vi "log analysis_gps.vi"() -> ()   [LabVIEW 2018] (continued)
0.0963,0.1004,5.0820,0f000001,0*f4eeef52\n\t", "INSPVAXA,USB3,0,47.5,FINESTEERING,2107,283761.800,02000000,471d,15824;INS_ALIGNMENT_COMPLETE,INS_RTKFIXED,37.37107239859,126.72171850723,8.1174,22.3000,-0.3618,-0.2694,0.0247,-0.806586304,0.185409278,212.363938082,0.4339,0.3017,0.5874,0.1136,0.0941,0.0830,0.0963,0.1004,5.0820,0f000001,0*fafaa8b9\n\t", "INSPVAXA,USB3,0,49.5,FINESTEERING,2107,283762.300,02000000,471d,15824;INS_ALIGNMENT_COMPLETE,INS_RTKFIXED,37.37107064339,126.72171694758,8.1181,22.3000,-0.3599,-0.2839,0.0222,-0.849299208,0.007344260,212.586929026,0.4338,0.3017,0.5881,0.1135,0.0943,0.0833,0.0964,0.1005,5.0831,0f000001,0*fde6b9b2\n\t", "DUALANTENNAHEADINGA,USB3,0,49.5,FINESTEERING,2107,283762.800,02000000,d426,15824;INSUFFICIENT_OBS,NONE,-1.000000000,0.000000000,0.000000000,0.0,0.000000000,0.000000000,\"631T\",11,2,2,2,04,00,20,00*344581c2\n\t", "INSPVAXA,USB3,0,49.5,FINESTEERING,2107,283763.300,02000000,471d,15824;INS_ALIGNMENT_COMPLETE,INS_RTKFIXED,37.37106722577,126.72171383567,8.1242,22.3000,-0.3707,-0.2828,0.0344,-0.877287415,-0.329953157,212.884392391,0.4341,0.3014,0.5889,0.1138,0.0946,0.0836,0.0965,0.1006,5.0839,0f000001,0*2db501e2\n\t", "INSPVAXA,USB3,0,49.5,FINESTEERING,2107,283763.800,02000000,471d,15824;INS_ALIGNMENT_COMPLETE,INS_RTKFIXED,37.37106551581,126.72171225128,8.1242,22.3000,-0.3497,-0.2822,0.0044,-0.644975976,-0.227422020,213.086413848,0.4341,0.3014,0.5889,0.1138,0.0946,0.0836,0.0965,0.1006,5.0839,0f000001,0*e7a51fd5\n\t", "INSPVAXA,USB3,0,50.0,FINESTEERING,2107,283764.300,02000000,471d,15824;INS_ALIGNMENT_COMPLETE,INS_RTKFIXED,37.37106379034,126.72171067271,8.1222,22.3000,-0.3531,-0.2829,0.0306,-0.817396197,-0.204433431,213.191870760,0.4344,0.3013,0.5897,0.1145,0.0953,0.0847,0.0966,0.1006,5.0845,0f000001,0*c35694b0\n\t", "INSPVAXA,USB3,0,50.0,FINESTEERING,2107,283764.800,02000000,471d,15824;INS_ALIGNMENT_COMPLETE,INS_RTKFIXED,37.37106210013,126.72170911188,8.1232,22.3000,-0.3512,-0.2846,0.0354,-0.878103846,0.017122797,213.188721115,0.4344,0.3013,0.5897,0.1145,0.0953,0.0847,0.0966,0.1006,5.0845,0f000001,0*f1b4f4ee\n\t", "INSPVAXA,USB3,0,48.5,FINESTEERING,2107,283765.300,02000000,471d,15824;INS_ALIGNMENT_COMPLETE,INS_RTKFIXED,37.37106036944,126.72170751159,8.1232,22.3000,-0.3518,-0.2906,0.0186,-0.822067301,0.160317962,213.455699651,0.4347,0.3015,0.5906,0.1149,0.0956,0.0855,0.0967,0.1007,5.0850,0f000001,0*76086230\n\t", "INSPVAXA,USB3,0,48.5,FINESTEERING,2107,283765.800,02000000,471d,15824;INS_ALIGNMENT_COMPLETE,INS_RTKFIXED,37.37105862901,126.72170591999,8.1228,22.3000,-0.3574,-0.2825,0.0115,-1.119312429,-0.040061536,213.743406523,0.4347,0.3015,0.5906,0.1149,0.0956,0.0855,0.0967,0.1007,5.0850,0f000001,0*ba4559e2\n\t", "INSPVAXA,USB3,0,49.5,FINESTEERING,2107,283766.300,02000000,471d,15824;INS_ALIGNMENT_COMPLETE,INS_RTKFIXED,37.37105695228,126.72170433159,8.1249,22.3000,-0.3688,-0.2983,0.0300,-0.908838629,-0.130495900,213.736346026,0.4351,0.3021,0.5917,0.1155,0.0961,0.0864,0.0968,0.1008,5.0859,0f000001,0*b472baf5\n\t", "DUALANTENNAHEADINGA,USB3,0,49.5,FINESTEERING,2107,283766.800,02000000,d426,15824;INSUFFICIENT_OBS,NONE,-1.000000000,0.000000000,0.000000000,0.0,0.000000000,0.000000000,\"631T\",12,2,2,2,04,00,20,00*fb02124e\n\t", "INSPVAXA,USB3,0,42.5,FINESTEERING,2107,283767.300,02000000,471d,15824;INS_ALIGNMENT_COMPLETE,INS_RTKFIXED,37.37105380440,126.72170132939,8.1248,22.3000,-0.4012,-0.3058,0.0222,-0.759918360,0.196787638,213.771684261,0.4356,0.3025,0.5930,0.1157,0.0960,0.0864,0.0969,0.1009,5.0866,0f000001,0*582355d6\n\t", "DUALANTENNAHEADINGA,USB3,0,42.5,FINESTEERING,2107,283767.800,02000000,d426,15824;INSUFFICIENT_OBS,NONE,-1.000000000,0.000000000,0.000000000,0.0,0.000000000,0.000000000,\"631T\",11,2,2,2,04,00,20,00*0d855270\n\t", "DUALANTENNAHEADINGA,USB3,0,49.5,FINESTEERING,2107,283768.300,02000000,d426,15824;INSUFFICIENT_OBS,NONE,-1.000000000,0.000000000,0.000000000,0.0,0.000000000,0.000000000,\"631T\",13,2,2,2,04,00,20,00*d65186ff\n\t", "INSPVAXA,USB3,0,49.5,FINESTEERING,2107,283768.800,02000000,471d,15824;INS_ALIGNMENT_COMPLETE,INS_RTKFIXED,37.37104867092,126.72169640975,8.1299,22.3000,-0.3630,-0.2854,0.0072,-0.696189759,0.706458627,213.919013530,0.4366,0.3037,0.5940,0.1145,0.0950,0.0854,0.0970,0.1010,5.0873,0f000001,0*a94daabe\n\t", "DUALANTENNAHEADINGA,USB3,0,49.0,FINESTEERING,2107,283769.300,02000000,d426,15824;INSUFFICIENT_OBS,NONE,-1.000000000,0.000000000,0.000000000,0.0,0.000000000,0.000000000,\"631T\",11,2,2,2,04,00,20,00*9a47621b\n\t", "INSPVAXA,USB3,0,49.0,FINESTEERING,2107,283769.800,02000000,471d,15824;INS_ALIGNMENT_COMPLETE,INS_RTKFIXED,37.37104525737,126.72169313095,8.1331,22.3000,-0.3548,-0.2589,0.0390,-0.749813070,0.572311932,213.822472384,0.4366,0.3042,0.5948,0.1140,0.0941,0.0845,0.0971,0.1011,5.0877,0f000001,0*7155f04b\n\t", "DUALANTENNAHEADINGA,USB3,0,51.5,FINESTEERING,2107,283770.300,02000000,d426,15824;INSUFFICIENT_OBS,NONE,-1.000000000,0.000000000,0.000000000,0.0,0.000000000,0.000000000,\"631T\",11,2,2,2,04,00,20,00*c0be82b5\n\t", "INSPVAXA,USB3,0,51.5,FINESTEERING,2107,283770.800,02000000,471d,15824;INS_ALIGNMENT_COMPLETE,INS_RTKFIXED,37.37104183450,126.72168993931,8.1368,22.3000,-0.3882,-0.2885,0.0511,-0.819164029,0.307516515,213.418856918,0.4363,0.3032,0.5950,0.1136,0.0937,0.0835,0.0972,0.1011,5.0881,0f000001,0*aed1500e\n\t", "INSPVAXA,USB3,0,48.5,FINESTEERING,2107,283771.300,02000000,471d,15824;INS_ALIGNMENT_COMPLETE,INS_RTKFIXED,37.37104011891,126.72168833768,8.1396,22.3000,-0.3597,-0.2669,0.0230,-0.734280477,0.363827676,213.144857898,0.4357,0.3026,0.5950,0.1131,0.0936,0.0827,0.0973,0.1011,5.0881,0f000001,0*55c65246\n\t", "DUALANTENNAHEADINGA,USB3,0,48.5,FINESTEERING,2107,283771.800,02000000,d426,15824;INSUFFICIENT_OBS,NONE,-1.000000000,0.000000000,0.000000000,0.0,0.000000000,0.000000000,\"631T\",12,2,2,2,04,00,20,00*ba5d6ed0\n\t", "DUALANTENNAHEADINGA,USB3,0,51.5,FINESTEERING,2107,283772.300,02000000,d426,15824;INSUFFICIENT_OBS,NONE,-1.000000000,0.000000000,0.000000000,0.0,0.000000000,0.000000000,\"631T\",10,2,2,2,04,00,20,00*ccec0b5f\n\t", "DUALANTENNAHEADINGA,USB3,0,51.5,FINESTEERING,2107,283772.800,02000000,d426,15824;INSUFFICIENT_OBS,NONE,-1.000000000,0.000000000,0.000000000,0.0,0.000000000,0.000000000,\"631T\",11,2,2,2,04,00,20,00*8e3ca933\n\t", "DUALANTENNAHEADINGA,USB3,0,51.0,FINESTEERING,2107,283773.300,02000000,d426,15824;INSUFFICIENT_OBS,NONE,-1.000000000,0.000000000,0.000000000,0.0,0.000000000,0.000000000,\"631T\",11,2,2,2,04,00,20,00*23ac6912\n\t", "DUALANTENNAHEADINGA,USB3,0,51.0,FINESTEERING,2107,283773.800,02000000,d426,15824;INSUFFICIENT_OBS,NONE,-1.000000000,0.000000000,0.000000000,0.0,0.000000000,0.000000000,\"631T\",11,2,2,2,04,00,20,00*b69e4b26\n\t", "DUALANTENNAHEADINGA,USB3,0,51.5,FINESTEERING,2107,283774.300,02000000,d426,15824;INSUFFICIENT_OBS,NONE,-1.000000000,0.000000000,0.000000000,0.0,0.000000000,0.000000000,\"631T\",10,2,2,2,04,00,20,00*7b4d17c8\n\t", "DUALANTENNAHEADINGA,USB3,0,51.5,FINESTEERING,2107,283774.800,02000000,d426,15824;INSUFFICIENT_OBS,NONE,-1.000000000,0.000000000,0.000000000,0.0,0.000000000,0.000000000,\"631T\",9,2,2,2,04,00,20,00*16022d9f\n\t", "INSPVAXA,USB3,0,52.5,FINESTEERING,2107,283775.300,02000000,471d,15824;INS_ALIGNMENT_COMPLETE,INS_RTKFIXED,37.37102638218,126.72167583323,8.1427,22.3000,-0.3501,-0.2557,0.0203,-0.739090378,0.635309618,211.720087902,0.4333,0.3004,0.5913,0.1131,0.0941,0.0802,0.0969,0.1010,5.0876,0f000001,0*37c46ea0\n\t", "INSPVAXA,USB3,0,52.5,FINESTEERING,2107,283775.800,02000000,471d,15824;INS_ALIGNMENT_COMPLETE,INS_RTKFIXED,37.37102462935,126.72167425219,8.1431,22.3000,-0.3596,-0.2647,0.0054,-0.635685510,0.684071691,211.684016338,0.4333,0.3004,0.5913,0.1131,0.0941,0.0802,0.0969,0.1010,5.0876,0f000001,0*5c9971d0\n\t", "DUALANTENNAHEADINGA,USB3,0,52.0,FINESTEERING,2107,283776.300,02000000,d426,15824;INSUFFICIENT_OBS,NONE,-1.000000000,0.000000000,0.000000000,0.0,0.000000000,0.000000000,\"631T\",11,2,2,2,04,00,20,00*8ea80302\n\t", "INSPVAXA,USB3,0,52.0,FINESTEERING,2107,283776.800,02000000,471d,15824;INS_ALIGNMENT_COMPLETE,INS_RTKFIXED,37.37102123220,126.72167119947,8.1450,22.3000,-0.3884,-0.2739,0.0352,-0.693294661,0.196719454,211.670955627,0.4336,0.3004,0.5905,0.1143,0.0952,0.0818,0.0967,0.1009,5.0864,0f000001,0*acb72d28\n\t", "DUALANTENNAHEADINGA,USB3,0,49.0,FINESTEERING,2107,283777.300,02000000,d426,15824;INSUFFICIENT_OBS,NONE,-1.000000000,0.000000000,0.000000000,0.0,0.000000000,0.000000000,\"631T\",10,2,2,2,04,00,20,00*dd4466ea\n\t", "INSPVAXA,USB3,0,49.0,FINESTEERING,2107,283777.800,02000000,471d,15824;INS_ALIGNMENT_COMPLETE,INS_RTKFIXED,37.37101775976,126.72166805938,8.1480,22.3000,-0.3623,-0.2643,0.0243,-0.564736999,0.528719086,211.738950079,0.4339,0.3012,0.5898,0.1140,0.0954,0.0814,0.0965,0.1008,5.0862,0f000001,0*673a0e61\n\t", "DUALANTENNAHEADINGA,USB3,0,52.0,FINESTEERING,2107,283778.300,02000000,d426,15824;INSUFFICIENT_OBS,NONE,-1.000000000,0.000000000,0.000000000,0.0,0.000000000,0.000000000,\"631T\",10,2,2,2,04,00,20,00*36c9b587\n\t", "DUALANTENNAHEADINGA,USB3,0,52.0,FINESTEERING,2107,283778.800,02000000,d426,15824;INSUFFICIENT_OBS,NONE,-1.000000000,0.000000000,0.000000000,0.0,0.000000000,0.000000000,\"631T\",12,2,2,2,04,00,20,00*d74f9142\n\t", "DUALANTENNAHEADINGA,USB3,0,51.0,FINESTEERING,2107,283779.300,02000000,d426,15824;INSUFFICIENT_OBS,NONE,-1.000000000,0.000000000,0.000000000,0.0,0.000000000,0.000000000,\"631T\",11,2,2,2,04,00,20,00*203e4aea\n\t", "DUALANTENNAHEADINGA,USB3,0,51.0,FINESTEERING,2107,283779.800,02000000,d426,15824;INSUFFICIENT_OBS,NONE,-1.000000000,0.000000000,0.000000000,0.0,0.000000000,0.000000000,\"631T\",11,2,2,2,04,00,20,00*b50c68de\n\t", "DUALANTENNAHEADINGA,USB3,0,51.0,FINESTEERING,2107,283780.300,02000000,d426,15824;INSUFFICIENT_OBS,NONE,-1.000000000,0.000000000,0.000000000,0.0,0.000000000,0.000000000,\"631T\",11,2,2,2,04,00,20,00*92abfb52\n\t", "DUALANTENNAHEADINGA,USB3,0,51.0,FINESTEERING,2107,283780.800,02000000,d426,15824;INSUFFICIENT_OBS,NONE,-1.000000000,0.000000000,0.000000000,0.0,0.000000000,0.000000000,\"631T\",13,2,2,2,04,00,20,00*732ddf97\n\t", "DUALANTENNAHEADINGA,USB3,0,48.5,FINESTEERING,2107,283781.300,02000000,d426,15824;INSUFFICIENT_OBS,NONE,-1.000000000,0.000000000,0.000000000,0.0,0.000000000,0.000000000,\"631T\",13,2,2,2,04,00,20,00*ffe25397\n\t", "DUALANTENNAHEADINGA,USB3,0,48.5,FINESTEERING,2107,283781.800,02000000,d426,15824;INSUFFICIENT_OBS,NONE,-1.000000000,0.000000000,0.000000000,0.0,0.000000000,0.000000000,\"631T\",13,2,2,2,04,00,20,00*6ad071a3\n\t", "DUALANTENNAHEADINGA,USB3,0,45.5,FINESTEERING,2107,283782.300,02000000,d426,15824;INSUFFICIENT_OBS,NONE,-1.000000000,0.000000000,0.000000000,0.0,0.000000000,0.000000000,\"631T\",14,2,2,2,04,00,20,00*b956e660\n\t", "DUALANTENNAHEADINGA,USB3,0,45.5,FINESTEERING,2107,283782.800,02000000,d426,15824;INSUFFICIENT_OBS,NONE,-1.000000000,0.000000000,0.000000000,0.0,0.000000000,0.000000000,\"631T\",15,2,2,2,04,00,20,00*fb86440c\n\t", "DUALANTENNAHEADINGA,USB3,0,46.5,FINESTEERING,2107,283783.300,02000000,d426,15824;INSUFFICIENT_OBS,NONE,-1.000000000,0.000000000,0.000000000,0.0,0.000000000,0.000000000,\"631T\",14,2,2,2,04,00,20,00*78439955\n\t", "DUALANTENNAHEADINGA,USB3,0,46.5,FINESTEERING,2107,283783.800,02000000,d426,15824;INSUFFICIENT_OBS,NONE,-1.000000000,0.000000000,0.000000000,0.0,0.000000000,0.000000000,\"631T\",13,2,2,2,04,00,20,00*a74f302a\n\t", "DUALANTENNAHEADINGA,USB3,0,48.5,FINESTEERING,2107,283784.300,02000000,d426,15824;INSUFFICIENT_OBS,NONE,-1.000000000,0.000000000,0.000000000,0.0,0.000000000,0.000000000,\"631T\",12,2,2,2,04,00,20,00*29c9c233\n\t", "INSPVAXA,USB3,0,48.5,FINESTEERING,2107,283784.850,02000000,471d,15824;INS_ALIGNMENT_COMPLETE,INS_RTKFIXED,37.37099341239,126.72164628694,8.2001,22.3000,-0.3345,-0.2518,0.0438,-0.619275773,0.409325340,212.136895574,0.4352,0.3052,0.5928,0.1145,0.0952,0.0844,0.0964,0.1005,5.0884,0f000001,0*694e34ff\n\t", "DUALANTENNAHEADINGA,USB3,0,51.5,FINESTEERING,2107,283785.300,02000000,d426,15824;INSUFFICIENT_OBS,NONE,-1.000000000,0.000000000,0.000000000,0.0,0.000000000,0.000000000,\"631T\",9,2,2,2,04,00,20,00*9cd19b46\n\t", "DUALANTENNAHEADINGA,USB3,0,51.5,FINESTEERING,2107,283785.800,02000000,d426,15824;INSUFFICIENT_OBS,NONE,-1.000000000,0.000000000,0.000000000,0.0,0.000000000,0.000000000,\"631T\",10,2,2,2,04,00,20,00*84c8ae0e\n\t", "DUALANTENNAHEADINGA,USB3,0,51.5,FINESTEERING,2107,283786.300,02000000,d426,15824;INSUFFICIENT_OBS,NONE,-1.000000000,0.000000000,0.000000000,0.0,0.000000000,0.000000000,\"631T\",10,2,2,2,04,00,20,00*a7928151\n\t", "DUALANTENNAHEADINGA,USB3,0,51.5,FINESTEERING,2107,283786.800,02000000,d426,15824;INSUFFICIENT_OBS,NONE,-1.000000000,0.000000000,0.000000000,0.0,0.000000000,0.000000000,\"631T\",10,2,2,2,04,00,20,00*32a0a365\n\t", "DUALANTENNAHEADINGA,USB3,0,51.5,FINESTEERING,2107,283787.300,02000000,d426,15824;INSUFFICIENT_OBS,NONE,-1.000000000,0.000000000,0.000000000,0.0,0.000000000,0.000000000,\"631T\",9,2,2,2,04,00,20,00*9711ff6c\n\t", "DUALANTENNAHEADINGA,USB3,0,51.5,FINESTEERING,2107,283787.800,02000000,d426,15824;INSUFFICIENT_OBS,NONE,-1.000000000,0.000000000,0.000000000,0.0,0.000000000,0.000000000,\"631T\",9,2,2,2,04,00,20,00*1a7949a4\n\t", "DUALANTENNAHEADINGA,USB3,0,51.0,FINESTEERING,2107,283788.300,02000000,d426,15824;INSUFFICIENT_OBS,NONE,-1.000000000,0.000000000,0.000000000,0.0,0.000000000,0.000000000,\"631T\",12,2,2,2,04,00,20,00*e9df57b1\n\t", "INSPVAXA,USB3,0,51.0,FINESTEERING,2107,283788.850,02000000,471d,15824;INS_ALIGNMENT_COMPLETE,INS_RTKFIXED,37.37097997438,126.72163399809,8.2319,22.3000,-0.3477,-0.2519,0.0287,-0.582557293,0.579304641,212.384981326,0.4350,0.3041,0.5941,0.1138,0.0947,0.0833,0.0968,0.1007,5.0940,0f000001,0*8f3b5f11\n\t", "DUALANTENNAHEADINGA,USB3,0,47.5,FINESTEERING,2107,283789.300,02000000,d426,15824;INSUFFICIENT_OBS,NONE,-1.000000000,0.000000000,0.000000000,0.0,0.000000000,0.000000000,\"631T\",11,2,2,2,04,00,20,00*211fe1b3\n\t", "DUALANTENNAHEADINGA,USB3,0,47.5,FINESTEERING,2107,283789.800,02000000,d426,15824;INSUFFICIENT_OBS,NONE,-1.000000000,0.000000000,0.000000000,0.0,0.000000000,0.000000000,\"631T\",11,2,2,2,04,00,20,00*b42dc387\n\t", "DUALANTENNAHEADINGA,USB3,0,48.0,FINESTEERING,2107,283791.300,02000000,d426,15824;INSUFFICIENT_OBS,NONE,-1.000000000,0.000000000,0.000000000,0.0,0.000000000,0.000000000,\"631T\",12,2,2,2,04,00,20,00*82188777\n\t", "DUALANTENNAHEADINGA,USB3,0,48.0,FINESTEERING,2107,283791.800,02000000,d426,15824;INSUFFICIENT_OBS,NONE,-1.000000000,0.000000000,0.000000000,0.0,0.000000000,0.000000000,\"631T\",11,2,2,2,04,00,20,00*b47c23ea\n\t", "DUALANTENNAHEADINGA,USB3,0,50.5,FINESTEERING,2107,283792.300,02000000,d426,15824;INSUFFICIENT_OBS,NONE,-1.000000000,0.000000000,0.000000000,0.0,0.000000000,0.000000000,\"631T\",10,2,2,2,04,00,20,00*50a5f0a4\n\t", "DUALANTENNAHEADINGA,USB3,0,50.5,FINESTEERING,2107,283792.800,02000000,d426,15824;INSUFFICIENT_OBS,NONE,-1.000000000,0.000000000,0.000000000,0.0,0.000000000,0.000000000,\"631T\",11,2,2,2,04,00,20,00*127552c8\n\t", "DUALANTENNAHEADINGA,USB3,0,51.0,FINESTEERING,2107,283793.300,02000000,d426,15824;INSUFFICIENT_OBS,NONE,-1.000000000,0.000000000,0.000000000,0.0,0.000000000,0.000000000,\"631T\",12,2,2,2,04,00,20,00*78f7c2e4\n\t", "DUALANTENNAHEADINGA,USB3,0,51.0,FINESTEERING,2107,283793.800,02000000,d426,15824;INSUFFICIENT_OBS,NONE,-1.000000000,0.000000000,0.000000000,0.0,0.000000000,0.000000000,\"631T\",12,2,2,2,04,00,20,00*edc5e0d0\n\t", "DUALANTENNAHEADINGA,USB3,0,49.0,FINESTEERING,2107,283794.300,02000000,d426,15824;INSUFFICIENT_OBS,NONE,-1.000000000,0.000000000,0.000000000,0.0,0.000000000,0.000000000,\"631T\",12,2,2,2,04,00,20,00*e795402f\n\t", "INSPVAXA,USB3,0,49.0,FINESTEERING,2107,283794.850,02000000,471d,15824;INS_ALIGNMENT_COMPLETE,INS_RTKFIXED,37.37095950999,126.72161470506,8.2822,22.3000,-0.3469,-0.2852,0.0349,-0.585483256,0.407743515,213.108220245,0.4436,0.3050,0.5933,0.1139,0.0939,0.0807,0.0967,0.1009,5.0986,0f000001,0*2d1ea958\n\t", "INSPVAXA,USB3,0,49.5,FINESTEERING,2107,283795.350,02000000,471d,15824;INS_ALIGNMENT_COMPLETE,INS_RTKFIXED,37.37095780554,126.72161308340,8.2866,22.3000,-0.3323,-0.2686,0.0234,-0.679981152,0.368181514,213.212479127,0.4428,0.3050,0.5925,0.1149,0.0952,0.0822,0.0966,0.1008,5.0998,0f000001,0*00d81367\n\t", "INSPVAXA,USB3,0,49.5,FINESTEERING,2107,283795.850,02000000,471d,15824;INS_ALIGNMENT_COMPLETE,INS_RTKFIXED,37.37095608366,126.72161143693,8.2891,22.3000,-0.3594,-0.2842,0.0245,-0.713487628,0.182586605,213.339171436,0.4428,0.3050,0.5925,0.1149,0.0952,0.0822,0.0966,0.1008,5.0998,0f000001,0*c6ad4823\n\t", "DUALANTENNAHEADINGA,USB3,0,49.0,FINESTEERING,2107,283796.300,02000000,d426,15824;INSUFFICIENT_OBS,NONE,-1.000000000,0.000000000,0.000000000,0.0,0.000000000,0.000000000,\"631T\",10,2,2,2,04,00,20,00*48914f6c\n\t", "DUALANTENNAHEADINGA,USB3,0,49.0,FINESTEERING,2107,283796.800,02000000,d426,15824;INSUFFICIENT_OBS,NONE,-1.000000000,0.000000000,0.000000000,0.0,0.000000000,0.000000000,\"631T\",11,2,2,2,04,00,20,00*0a41ed00\n\t", "DUALANTENNAHEADINGA,USB3,0,48.0,FINESTEERING,2107,283797.300,02000000,d426,15824;INSUFFICIENT_OBS,NONE,-1.000000000,0.000000000,0.000000000,0.0,0.000000000,0.000000000,\"631T\",9,2,2,2,04,00,20,00*6eb18c36\n\t", "INSPVAXA,USB3,0,48.0,FINESTEERING,2107,283797.850,02000000,471d,15824;INS_ALIGNMENT_COMPLETE,INS_RTKFIXED,37.37094930309,126.72160503752,8.2955,22.3000,-0.3503,-0.2634,0.0529,-0.883186329,0.520080869,213.088491004,0.4411,0.3046,0.5913,0.1142,0.0943,0.0813,0.0964,0.1007,5.1027,0f000001,0*48f5b9d5\n\t", "INSPVAXA,USB3,0,49.0,FINESTEERING,2107,283798.350,02000000,471d,15824;INS_ALIGNMENT_COMPLETE,INS_RTKFIXED,37.37094758221,126.72160345161,8.2970,22.3000,-0.3412,-0.2718,0.0078,-0.914982757,0.563532135,212.970746608,0.4404,0.3047,0.5910,0.1139,0.0940,0.0809,0.0964,0.1006,5.1042,0f000001,0*9baeb022\n\t", "DUALANTENNAHEADINGA,USB3,0,49.0,FINESTEERING,2107,283798.800,02000000,d426,15824;INSUFFICIENT_OBS,NONE,-1.000000000,0.000000000,0.000000000,0.0,0.000000000,0.000000000,\"631T\",12,2,2,2,04,00,20,00*c6945d74\n\t", "DUALANTENNAHEADINGA,USB3,0,45.5,FINESTEERING,2107,283799.300,02000000,d426,15824;INSUFFICIENT_OBS,NONE,-1.000000000,0.000000000,0.000000000,0.0,0.000000000,0.000000000,\"631T\",11,2,2,2,04,00,20,00*16f4fe8f\n\t", "INSPVAXA,USB3,0,49.0,FINESTEERING,2107,283800.350,02000000,471d,15824;INS_ALIGNMENT_COMPLETE,INS_RTKFIXED,37.37094091423,126.72159737065,8.3045,22.3000,-0.3067,-0.2479,0.0203,-0.819842443,0.191371077,212.561808426,0.4393,0.3042,0.5904,0.1136,0.0943,0.0803,0.0963,0.1005,5.1071,0f000001,0*87713df7\n\t", "INSPVAXA,USB3,0,49.0,FINESTEERING,2107,283800.850,02000000,471d,15824;INS_ALIGNMENT_COMPLETE,INS_RTKFIXED,37.37093917106,126.72159578711,8.3082,22.3000,-0.3234,-0.2591,0.0222,-0.646837907,0.336367436,212.664833979,0.4393,0.3042,0.5904,0.1136,0.0943,0.0803,0.0963,0.1005,5.1071,0f000001,0*a47e26e8\n\t", "INSPVAXA,USB3,0,42.0,FINESTEERING,2107,283801.350,02000000,471d,15824;INS_ALIGNMENT_COMPLETE,INS_RTKFIXED,37.37093749345,126.72159425291,8.3098,22.3000,-0.3764,-0.2836,0.0471,-0.642147741,0.485055187,212.666460459,0.4391,0.3035,0.5903,0.1145,0.0947,0.0815,0.0963,0.1005,5.1074,0f000001,0*cfb387f2\n\t", "INSPVAXA,USB3,0,42.0,FINESTEERING,2107,283801.850,02000000,471d,15824;INS_ALIGNMENT_COMPLETE,INS_RTKFIXED,37.37093581786,126.72159270156,8.3102,22.3000,-0.3221,-0.2542,0.0038,-0.637890069,0.520458025,212.703870431,0.4391,0.3035,0.5903,0.1145,0.0947,0.0815,0.0963,0.1005,5.1074,0f000001,0*42dc58c1\n\t", "INSPVAXA,USB3,0,48.0,FINESTEERING,2107,283802.350,02000000,471d,15824;INS_ALIGNMENT_COMPLETE,INS_RTKFIXED,37.37093409830,126.72159111901,8.3142,22.3000,-0.3534,-0.2655,0.0351,-0.709498391,0.532234116,212.787033062,0.4389,0.3043,0.5904,0.1141,0.0944,0.0812,0.0962,0.1004,5.1086,0f000001,0*ada231a9\n\t", "INSPVAXA,USB3,0,48.0,FINESTEERING,2107,283802.850,02000000,471d,15824;INS_ALIGNMENT_COMPLETE,INS_RTKFIXED,37.37093238773,126.72158954092,8.3176,22.3000,-0.3340,-0.2726,0.0399,-0.642602467,0.406541705,212.810181353,0.4389,0.3043,0.5904,0.1141,0.0944,0.0812,0.0962,0.1004,5.1086,0f000001,0*fb1d3214\n\t", "INSPVAXA,USB3,0,50.0,FINESTEERING,2107,283803.350,02000000,471d,15824;INS_ALIGNMENT_COMPLETE,INS_RTKFIXED,37.37093069995,126.72158798195,8.3220,22.3000,-0.3417,-0.2608,0.0173,-0.694649524,0.610927882,212.865796142,0.4386,0.3050,0.5904,0.1147,0.0949,0.0821,0.0962,0.1004,5.1101,0f000001,0*664f4704\n\t", "INSPVAXA,USB3,0,50.0,FINESTEERING,2107,283803.850,02000000,471d,15824;INS_ALIGNMENT_COMPLETE,INS_RTKFIXED,37.37092900254,126.72158638121,8.3251,22.3000,-0.3538,-0.2865,0.0254,-0.433488286,0.440900980,212.995869774,0.4386,0.3050,0.5904,0.1147,0.0949,0.0821,0.0962,0.1004,5.1101,0f000001,0*a84e9ea6\n\t", "INSPVAXA,USB3,0,48.0,FINESTEERING,2107,283804.350,02000000,471d,15824;INS_ALIGNMENT_COMPLETE,INS_RTKFIXED,37.37092729858,126.72158475162,8.3262,22.3000,-0.3346,-0.2736,0.0337,-0.198500988,0.485164152,213.066525624,0.4382,0.3051,0.5905,0.1141,0.0944,0.0817,0.0962,0.1004,5.1114,0f000001,0*c4e8da54\n\t", "INSPVAXA,USB3,0,48.0,FINESTEERING,2107,283804.850,02000000,471d,15824;INS_ALIGNMENT_COMPLETE,INS_RTKFIXED,37.37092559356,126.72158315411,8.3286,22.3000,-0.3344,-0.2698,0.0356,-0.560548188,0.428951869,213.152040125,0.4382,0.3051,0.5905,0.1141,0.0944,0.0817,0.0962,0.1004,5.1114,0f000001,0*865f3348\n\t", "INSPVAXA,USB3,0,50.5,FINESTEERING,2107,283805.350,02000000,471d,15824;INS_ALIGNMENT_COMPLETE,INS_RTKFIXED,37.37092390925,126.72158151800,8.3310,22.3000,-0.3577,-0.2766,0.0312,-0.244742363,0.378624826,213.232619206,0.4377,0.3050,0.5905,0.1137,0.0939,0.0814,0.0962,0.1003,5.1129,0f000001,0*93a69a58\n\t", "INSPVAXA,USB3,0,51.0,FINESTEERING,2107,283806.350,02000000,471d,15824;INS_ALIGNMENT_COMPLETE,INS_RTKFIXED,37.37092052937,126.72157829690,8.3375,22.3000,-0.3440,-0.2795,0.0245,-0.465963804,0.886312303,213.254279307,0.4369,0.3047,0.5904,0.1133,0.0936,0.0810,0.0962,0.1003,5.1143,0f000001,0*ac9069ee\n\t", "INSPVAXA,USB3,0,51.0,FINESTEERING,2107,283806.850,02000000,471d,15824;INS_ALIGNMENT_COMPLETE,INS_RTKFIXED,37.37091879437,126.72157664668,8.3407,22.3000,-0.3462,-0.2861,0.0240,-0.657037721,0.825600095,213.429652251,0.4369,0.3047,0.5904,0.1133,0.0936,0.0810,0.0962,0.1003,5.1143,0f000001,0*17c14289\n\t", "INSPVAXA,USB3,0,48.5,FINESTEERING,2107,283807.850,02000000,471d,15824;INS_ALIGNMENT_COMPLETE,INS_RTKFIXED,37.37091541659,126.72157338154,8.3525,22.3000,-0.3441,-0.2744,0.0198,-0.559398750,0.972716137,213.514077628,0.4363,0.3044,0.5901,0.1131,0.0934,0.0806,0.0963,0.1003,5.1156,0f000001,0*75ff1fc6\n\t", "INSPVAXA,USB3,0,44.5,FINESTEERING,2107,283808.350,02000000,471d,15824;INS_ALIGNMENT_COMPLETE,INS_RTKFIXED,37.37091372939,126.72157175918,8.3549,22.3000,-0.3553,-0.2831,0.0286,-0.709577121,1.164612328,213.658250013,0.4360,0.3038,0.5897,0.1132,0.0934,0.0803,0.0963,0.1003,5.1169,0f000001,0*14793968\n\t", "INSPVAXA,USB3,0,44.5,FINESTEERING,2107,283808.850,02000000,471d,15824;INS_ALIGNMENT_COMPLETE,INS_RTKFIXED,37.37091204717,126.72157012311,8.3593,22.3000,-0.3351,-0.2933,0.0335,-0.548646333,0.899552178,213.508678338,0.4360,0.3038,0.5897,0.1132,0.0934,0.0803,0.0963,0.1003,5.1169,0f000001,0*e79048d5\n\t", "INSPVAXA,USB3,0,46.0,FINESTEERING,2107,283809.350,02000000,471d,15824;INS_ALIGNMENT_COMPLETE,INS_RTKFIXED,37.37091031450,126.72156845279,8.3650,22.3000,-0.3479,-0.2887,0.0292,-0.530979071,0.488041271,213.615691599,0.4360,0.3037,0.5892,0.1129,0.0933,0.0800,0.0963,0.1003,5.1177,0f000001,0*4685a971\n\t", "INSPVAXA,USB3,0,46.0,FINESTEERING,2107,283809.850,02000000,471d,15824;INS_ALIGNMENT_COMPLETE,INS_RTKFIXED,37.37090862475,126.72156681870,8.3704,22.3000,-0.3507,-0.2732,0.0187,-0.627436643,0.484815097,213.766429758,0.4360,0.3037,0.5892,0.1129,0.0933,0.0800,0.0963,0.1003,5.1177,0f000001,0*042f58f5\n\t", "INSPVAXA,USB3,0,46.5,FINESTEERING,2107,283810.350,02000000,471d,15824;INS_ALIGNMENT_COMPLETE,INS_RTKFIXED,37.37090694651,126.72156520391,8.3753,22.3000,-0.3165,-0.2719,0.0394,-0.596255769,0.780970899,213.702239240,0.4358,0.3031,0.5888,0.1129,0.0933,0.0798,0.0963,0.1003,5.1187,0f000001,0*196b83f4\n\t", "INSPVAXA,USB3,0,46.5,FINESTEERING,2107,283810.850,02000000,471d,15824;INS_ALIGNMENT_COMPLETE,INS_RTKFIXED,37.37090525382,126.72156361193,8.3794,22.3000,-0.3598,-0.2713,0.0249,-0.973711193,1.074767761,213.656129114,0.4358,0.3031,0.5888,0.1129,0.0933,0.0798,0.0963,0.1003,5.1187,0f000001,0*60ffddbf\n\t", "INSPVAXA,USB3,0,49.0,FINESTEERING,2107,283811.350,02000000,471d,15824;INS_ALIGNMENT_COMPLETE,INS_RTKFIXED,37.37090357920,126.72156200390,8.3845,22.3000,-0.3442,-0.2800,0.0256,-0.979609219,0.857511693,213.501334190,0.4355,0.3025,0.5885,0.1131,0.0935,0.0796,0.0962,0.1002,5.1194,0f000001,0*aa11bf3c\n\t", "INSPVAXA,USB3,0,49.0,FINESTEERING,2107,283811.850,02000000,471d,15824;INS_ALIGNMENT_COMPLETE,INS_RTKFIXED,37.37090187370,126.72156034536,8.3910,22.3000,-0.3251,-0.2819,0.0474,-0.722859580,0.747515698,213.305789576,0.4355,0.3025,0.5885,0.1131,0.0935,0.0796,0.0962,0.1002,5.1194,0f000001,0*3fd13bdf\n\t", "INSPVAXA,USB3,0,49.5,FINESTEERING,2107,283812.350,02000000,471d,15824;INS_ALIGNMENT_COMPLETE,INS_RTKFIXED,37.37090016195,126.72155872579,8.3941,22.3000,-0.3301,-0.2714,0.0230,-0.816861765,0.807045897,213.365991854,0.4358,0.3019,0.5880,0.1129,0.0935,0.0794,0.0962,0.1002,5.1192,0f000001,0*4c65b004\n\t", "INSPVAXA,USB3,0,49.5,FINESTEERING,2107,283812.850,02000000,471d,15824;INS_ALIGNMENT_COMPLETE,INS_RTKFIXED,37.37089850948,126.72155716436,8.4007,22.3000,-0.3466,-0.2674,0.0245,-1.010459105,1.203472326,213.239594675,0.4358,0.3019,0.5880,0.1129,0.0935,0.0794,0.0962,0.1002,5.1192,0f000001,0*1434da4d\n\t", "INSPVAXA,USB3,0,49.0,FINESTEERING,2107,283813.350,02000000,471d,15824;INS_ALIGNMENT_COMPLETE,INS_RTKFIXED,37.37089680632,126.72155557603,8.4063,22.3000,-0.3291,-0.2810,0.0480,-0.955572188,1.123844377,213.096084553,0.4352,0.3013,0.5874,0.1129,0.0933,0.0793,0.0961,0.1001,5.1186,0f000001,0*817699e2\n\t", "INSPVAXA,USB3,0,49.0,FINESTEERING,2107,283813.850,02000000,471d,15824;INS_ALIGNMENT_COMPLETE,INS_RTKFIXED,37.37089510360,126.72155399997,8.4119,22.3000,-0.3389,-0.2720,0.0269,-0.936574530,0.986776176,213.030169664,0.4352,0.3013,0.5874,0.1129,0.0933,0.0793,0.0961,0.1001,5.1186,0f000001,0*5c3995b3\n\t", "INSPVAXA,USB3,0,49.5,FINESTEERING,2107,283814.350,02000000,471d,15824;INS_ALIGNMENT_COMPLETE,INS_RTKFIXED,37.37089337891,126.72155240702,8.4168,22.3000,-0.3379,-0.2725,0.0259,-0.990897752,0.543543172,212.990799562,0.4348,0.3013,0.5869,0.1127,0.0935,0.0792,0.0960,0.1000,5.1178,0f000001,0*80d17f12\n\t", "INSPVAXA,USB3,0,49.0,FINESTEERING,2107,283815.350,02000000,471d,15824;INS_ALIGNMENT_COMPLETE,INS_RTKFIXED,37.37088996706,126.72154929258,8.4245,22.3000,-0.3434,-0.2641,0.0250,-1.164432895,0.561258596,212.864234070,0.4342,0.3009,0.5863,0.1129,0.0938,0.0795,0.0959,0.1000,5.1167,0f000001,0*c7d2a868\n\t", "INSPVAXA,USB3,0,49.0,FINESTEERING,2107,283815.850,02000000,471d,15824;INS_ALIGNMENT_COMPLETE,INS_RTKFIXED,37.37088825034,126.72154772822,8.4276,22.3000,-0.3370,-0.2619,0.0268,-1.087119592,0.609799872,212.870793479,0.4342,0.3009,0.5863,0.1129,0.0938,0.0795,0.0959,0.1000,5.1167,0f000001,0*f57586d5\n\t", "INSPVAXA,USB3,0,45.5,FINESTEERING,2107,283816.350,02000000,471d,15824;INS_ALIGNMENT_COMPLETE,INS_RTKFIXED,37.37088648339,126.72154610950,8.4307,22.3000,-0.3394,-0.2623,0.0227,-0.831042768,0.509272652,212.987067657,0.4339,0.3006,0.5859,0.1127,0.0936,0.0794,0.0958,0.0999,5.1151,0f000001,0*c540a699\n\t", "INSPVAXA,USB3,0,45.5,FINESTEERING,2107,283816.850,02000000,471d,15824;INS_ALIGNMENT_COMPLETE,INS_RTKFIXED,37.37088478874,126.72154457975,8.4339,22.3000,-0.3715,-0.2876,0.0149,-0.938105772,0.365449923,213.063297584,0.4339,0.3006,0.5859,0.1127,0.0936,0.0794,0.0958,0.0999,5.1151,0f000001,0*840abd00\n\t", "INSPVAXA,USB3,0,46.5,FINESTEERING,2107,283817.350,02000000,471d,15824;INS_ALIGNMENT_COMPLETE,INS_RTKFIXED,37.37088307773,126.72154302879,8.4374,22.3000,-0.3594,-0.2773,0.0287,-0.958522380,0.243905829,212.991264938,0.4341,0.3007,0.5858,0.1132,0.0942,0.0801,0.0958,0.0999,5.1140,0f000001,0*fa6ad0ef\n\t", "INSPVAXA,USB3,0,46.5,FINESTEERING,2107,283817.850,02000000,471d,15824;INS_ALIGNMENT_COMPLETE,INS_RTKFIXED,37.37088132753,126.72154143045,8.4401,22.3000,-0.3278,-0.2536,0.0246,-0.732605001,0.589727641,213.014456450,0.4341,0.3007,0.5858,0.1132,0.0942,0.0801,0.0958,0.0999,5.1140,0f000001,0*274257ec\n\t", "INSPVAXA,USB3,0,42.0,FINESTEERING,2107,283818.350,02000000,471d,15824;INS_ALIGNMENT_COMPLETE,INS_RTKFIXED,37.37087991199,126.72154012021,8.4416,22.3000,-0.1368,-0.1470,0.0384,-0.668714112,0.493381563,212.999632348,0.4348,0.3009,0.5860,0.1136,0.0943,0.0809,0.0957,0.0999,5.1129,0f000001,0*1003161e\n\t", "INSPVAXA,USB3,0,42.0,FINESTEERING,2107,283818.850,02000000,471d,15824;INS_ALIGNMENT_COMPLETE,INS_RTKFIXED,37.37087810564,126.72153855101,8.4445,22.3000,-0.4167,-0.3108,0.0271,-0.967030857,0.764287443,212.987620648,0.4348,0.3009,0.5860,0.1136,0.0943,0.0809,0.0957,0.0999,5.1129,0f000001,0*cade7f0f\n\t", "INSPVAXA,USB3,0,48.0,FINESTEERING,2107,283819.850,02008000,471d,15824;INS_ALIGNMENT_COMPLETE,INS_RTKFIXED,37.37087469725,126.72153545428,8.4519,22.3000,-0.3206,-0.2482,0.0337,-0.732742938,0.483764401,213.124733025,0.4356,0.3015,0.5865,0.1140,0.0945,0.0816,0.0957,0.0999,5.1129,0f000001,0*fd809d66\n\t", "INSPVAXA,USB3,0,50.0,FINESTEERING,2107,283820.350,02008000,471d,15824;INS_ALIGNMENT_COMPLETE,INS_RTKFIXED,37.37087296887,126.72153391310,8.4559,22.3000,-0.3682,-0.2755,0.0355,-0.960553377,0.385725607,213.158574943,0.4360,0.3020,0.5871,0.1135,0.0940,0.0814,0.0957,0.0998,5.1132,0f000001,0*75b28094\n\t", "INSPVAXA,USB3,0,50.0,FINESTEERING,2107,283820.850,02008000,471d,15824;INS_ALIGNMENT_COMPLETE,INS_RTKFIXED,37.37087124768,126.72153233501,8.4599,22.3000,-0.3422,-0.2623,0.0223,-0.701545718,0.294421215,213.284375134,0.4360,0.3020,0.5871,0.1135,0.0940,0.0814,0.0957,0.0998,5.1132,0f000001,0*60222fab\n\t", "INSPVAXA,USB3,0,47.5,FINESTEERING,2107,283822.350,02008000,471d,15824;INS_ALIGNMENT_COMPLETE,INS_RTKFIXED,37.37086605631,126.72152760376,8.4704,22.3000,-0.3621,-0.2743,0.0261,-0.283958225,0.746560845,213.501890375,0.4357,0.3020,0.5877,0.1128,0.0932,0.0807,0.0958,0.0999,5.1149,0f000001,0*0669f83a\n\t", "INSPVAXA,USB3,0,47.5,FINESTEERING,2107,283822.850,02008000,471d,15824;INS_ALIGNMENT_COMPLETE,INS_RTKFIXED,37.37086430536,126.72152600341,8.4729,22.3000,-0.3685,-0.2624,0.0208,-0.369026169,0.243772602,213.702415244,0.4357,0.3020,0.5877,0.1128,0.0932,0.0807,0.0958,0.0999,5.1149,0f000001,0*05a2b3f5\n\t", "INSPVAXA,USB3,0,51.5,FINESTEERING,2107,283823.350,02000000,471d,15824;INS_ALIGNMENT_COMPLETE,INS_RTKFIXED,37.37086260441,126.72152443604,8.4782,22.3000,-0.3582,-0.2656,0.0432,-0.497136063,0.605287722,213.732183523,0.4353,0.3025,0.5877,0.1126,0.0930,0.0805,0.0959,0.0999,5.1164,0f000001,0*99f3cfc8\n\t", "INSPVAXA,USB3,0,50.0,FINESTEERING,2107,283826.350,02000000,471d,15824;INS_ALIGNMENT_COMPLETE,INS_RTKFIXED,37.37085224696,126.72151466397,8.5036,22.3000,-0.3609,-0.2791,0.0409,-0.133797163,0.866362629,214.216095146,0.4345,0.3034,0.5878,0.1129,0.0936,0.0804,0.0960,0.1000,5.1194,0f000001,0*7d577a89\n\t", "INSPVAXA,USB3,0,50.0,FINESTEERING,2107,283826.850,02000000,471d,15824;INS_ALIGNMENT_COMPLETE,INS_RTKFIXED,37.37085047497,126.72151297785,8.5076,22.3000,-0.3736,-0.2676,0.0140,-0.059092232,0.621746076,214.361721087,0.4345,0.3034,0.5878,0.1129,0.0936,0.0804,0.0960,0.1000,5.1194,0f000001,0*1a2aa4a2\n\t", "INSPVAXA,USB3,0,47.0,FINESTEERING,2107,283828.850,02000000,471d,15824;INS_ALIGNMENT_COMPLETE,INS_RTKFIXED,37.37084355919,126.72150637181,8.5210,22.3000,-0.3615,-0.2654,0.0256,-0.407156053,0.613221489,214.165441320,0.4336,0.3030,0.5876,0.1126,0.0934,0.0800,0.0960,0.1000,5.1212,0f000001,0*2be625c6\n\t", "INSPVAXA,USB3,0,49.5,FINESTEERING,2107,283833.350,02000000,471d,15824;INS_ALIGNMENT_COMPLETE,INS_RTKFIXED,37.37082814557,126.72149191799,8.5253,22.3000,-0.3988,-0.2653,0.0143,-0.599400887,0.523128391,213.276992929,0.4351,0.3016,0.5901,0.1136,0.0943,0.0827,0.0961,0.1001,5.1237,0f000001,0*dafc27db\n\t", "INSPVAXA,USB3,0,51.5,FINESTEERING,2107,283847.900,02000000,471d,15824;INS_ALIGNMENT_COMPLETE,INS_RTKFIXED,37.37077798648,126.72144617612,8.6277,22.3000,-0.3813,-0.2770,0.0286,-0.218735739,0.822253725,211.859941742,0.4334,0.3030,0.5894,0.1137,0.0946,0.0820,0.0959,0.1000,5.1292,0f000001,0*a6b72ce6\n\t", "INSPVAXA,USB3,0,50.5,FINESTEERING,2107,283849.400,02000000,471d,15824;INS_ALIGNMENT_COMPLETE,INS_RTKFIXED,37.37077272118,126.72144151665,8.6465,22.3000,-0.4175,-0.3003,0.0168,-0.333999296,0.525608406,211.832287674,0.4333,0.3042,0.5899,0.1136,0.0946,0.0824,0.0960,0.1001,5.1298,0f000001,0*7349f925\n\t", "INSPVAXA,USB3,0,41.0,FINESTEERING,2107,283850.900,02000000,471d,15824;INS_ALIGNMENT_COMPLETE,INS_RTKFIXED,37.37076749535,126.72143686208,8.6606,22.3000,-0.3847,-0.2816,0.0281,-0.406598384,0.513432483,212.015462221,0.4333,0.3045,0.5903,0.1132,0.0939,0.0820,0.0961,0.1001,5.1303,0f000001,0*8e06507b\n\t", "INSPVAXA,USB3,0,51.0,FINESTEERING,2107,283854.400,02000000,471d,15824;INS_ALIGNMENT_COMPLETE,INS_RTKFIXED,37.37075554514,126.72142617070,8.7046,22.3000,-0.3702,-0.2734,0.0406,-0.208946462,1.069935168,212.200844813,0.4356,0.3041,0.5961,0.1134,0.0944,0.0821,0.0963,0.1002,5.1349,0f000001,0*eaf32da8\n\t", "INSPVAXA,USB3,0,52.5,FINESTEERING,2107,283855.400,02000000,471d,15824;INS_ALIGNMENT_COMPLETE,INS_RTKFIXED,37.37075208909,126.72142312545,8.7152,22.3000,-0.3888,-0.2785,0.0279,-0.502124880,0.807271282,212.351278454,0.4348,0.3040,0.5953,0.1133,0.0940,0.0816,0.0963,0.1002,5.1361,0f000001,0*26b77d4e\n\t", "INSPVAXA,USB3,0,52.5,FINESTEERING,2107,283855.900,02000000,471d,15824;INS_ALIGNMENT_COMPLETE,INS_RTKFIXED,37.37075038942,126.72142158334,8.7226,22.3000,-0.3755,-0.2603,0.0501,-0.282397240,0.801872583,212.409267402,0.4348,0.3040,0.5953,0.1133,0.0940,0.0816,0.0963,0.1002,5.1361,0f000001,0*7c1b1b61\n\t", "INSPVAXA,USB3,0,53.5,FINESTEERING,2107,283856.400,02000000,471d,15824;INS_ALIGNMENT_COMPLETE,INS_RTKFIXED,37.37074865373,126.72142004246,8.7267,22.3000,-0.3704,-0.2786,0.0171,-0.353111883,0.600799682,212.485026381,0.4344,0.3035,0.5945,0.1128,0.0938,0.0812,0.0963,0.1002,5.1372,0f000001,0*81e7853e\n\t", "INSPVAXA,USB3,0,53.5,FINESTEERING,2107,283856.900,02000000,471d,15824;INS_ALIGNMENT_COMPLETE,INS_RTKFIXED,37.37074693319,126.72141850353,8.7310,22.3000,-0.3735,-0.2746,0.0382,-0.533241802,0.632806035,212.664304846,0.4344,0.3035,0.5945,0.1128,0.0938,0.0812,0.0963,0.1002,5.1372,0f000001,0*a05af5ad\n\t", "INSPVAXA,USB3,0,49.5,FINESTEERING,2107,283857.400,02000000,471d,15824;INS_ALIGNMENT_COMPLETE,INS_RTKFIXED,37.37074522542,126.72141694545,8.7353,22.3000,-0.3672,-0.2584,0.0083,-0.503263302,0.873939693,212.796225094,0.4338,0.3028,0.5936,0.1126,0.0936,0.0808,0.0963,0.1002,5.1384,0f000001,0*83ef516a\n\t", "INSPVAXA,USB3,0,48.5,FINESTEERING,2107,283858.400,02000000,471d,15824;INS_ALIGNMENT_COMPLETE,INS_RTKFIXED,37.37074181137,126.72141381926,8.7415,22.3000,-0.3728,-0.3056,0.0242,-0.533104830,1.057002190,212.963002885,0.4334,0.3023,0.5928,0.1134,0.0944,0.0817,0.0962,0.1002,5.1397,0f000001,0*eea1e126\n\t", "INSPVAXA,USB3,0,48.5,FINESTEERING,2107,283858.900,02000000,471d,15824;INS_ALIGNMENT_COMPLETE,INS_RTKFIXED,37.37074011417,126.72141223787,8.7461,22.3000,-0.3747,-0.2786,0.0449,-0.561180315,0.752123246,213.105436806,0.4334,0.3023,0.5928,0.1134,0.0944,0.0817,0.0962,0.1002,5.1397,0f000001,0*c4922269\n\t", "INSPVAXA,USB3,0,46.0,FINESTEERING,2107,283859.900,02000000,471d,15824;INS_ALIGNMENT_COMPLETE,INS_RTKFIXED,37.37073667123,126.72140904709,8.7547,22.3000,-0.3866,-0.2889,0.0316,-0.473578727,0.831151381,213.327049680,0.4335,0.3024,0.5921,0.1137,0.0949,0.0823,0.0962,0.1002,5.1407,0f000001,0*c02ad3f9\n\t", "INSPVAXA,USB3,0,48.5,FINESTEERING,2107,283860.400,02000000,471d,15824;INS_ALIGNMENT_COMPLETE,INS_RTKFIXED,37.37073499313,126.72140747004,8.7594,22.3000,-0.3720,-0.2575,0.0488,-0.469904775,1.004834179,213.445822894,0.4337,0.3023,0.5918,0.1139,0.0949,0.0827,0.0962,0.1002,5.1415,0f000001,0*acdd0918\n\t", "INSPVAXA,USB3,0,51.0,FINESTEERING,2107,283861.400,02000000,471d,15824;INS_ALIGNMENT_COMPLETE,INS_RTKFIXED,37.37073158735,126.72140425235,8.7667,22.3000,-0.3807,-0.2830,0.0264,-0.516210475,0.946045536,213.526350535,0.4337,0.3025,0.5918,0.1135,0.0942,0.0822,0.0962,0.1002,5.1424,0f000001,0*0628bfaf\n\t", "INSPVAXA,USB3,0,51.0,FINESTEERING,2107,283861.900,02000000,471d,15824;INS_ALIGNMENT_COMPLETE,INS_RTKFIXED,37.37072989036,126.72140267058,8.7698,22.3000,-0.3805,-0.2823,0.0328,-0.596244967,0.822145304,213.518686009,0.4337,0.3025,0.5918,0.1135,0.0942,0.0822,0.0962,0.1002,5.1424,0f000001,0*59f9b731\n\t", "INSPVAXA,USB3,0,53.5,FINESTEERING,2107,283862.900,02000000,471d,15824;INS_ALIGNMENT_COMPLETE,INS_RTKFIXED,37.37072646005,126.72139945545,8.7731,22.3000,-0.3733,-0.2791,0.0108,-0.480391317,0.493865630,213.689633604,0.4337,0.3029,0.5918,0.1135,0.0944,0.0825,0.0962,0.1002,5.1434,0f000001,0*a4999ec0\n\t", "INSPVAXA,USB3,0,51.0,FINESTEERING,2107,283863.400,02000000,471d,15824;INS_ALIGNMENT_COMPLETE,INS_RTKFIXED,37.37072475302,126.72139787824,8.7760,22.3000,-0.3764,-0.2596,0.0258,-0.739706001,0.670082501,213.669288600,0.4337,0.3025,0.5920,0.1136,0.0946,0.0829,0.0962,0.1002,5.1442,0f000001,0*2644d37e\n\t", "INSPVAXA,USB3,0,51.0,FINESTEERING,2107,283863.900,02000000,471d,15824;INS_ALIGNMENT_COMPLETE,INS_RTKFIXED,37.37072304752,126.72139625186,8.7774,22.3000,-0.3739,-0.2776,0.0095,-0.592048813,0.512858397,213.725097807,0.4337,0.3025,0.5920,0.1136,0.0946,0.0829,0.0962,0.1002,5.1442,0f000001,0*9580d57a\n\t", "INSPVAXA,USB3,0,48.5,FINESTEERING,2107,283864.400,02000000,471d,15824;INS_ALIGNMENT_COMPLETE,INS_RTKFIXED,37.37072134638,126.72139464126,8.7780,22.3000,-0.3662,-0.2725,0.0206,-0.511623152,0.752820747,213.729098110,0.4338,0.3024,0.5923,0.1139,0.0949,0.0834,0.0963,0.1002,5.1449,0f000001,0*0ef3aee0\n\t", "INSPVAXA,USB3,0,48.5,FINESTEERING,2107,283864.900,02000000,471d,15824;INS_ALIGNMENT_COMPLETE,INS_RTKFIXED,37.37071966406,126.72139308465,8.7791,22.3000,-0.2990,-0.2177,0.0217,-0.848822059,0.608273081,213.821443632,0.4338,0.3024,0.5923,0.1139,0.0949,0.0834,0.0963,0.1002,5.1449,0f000001,0*1bce49ab\n\t", "INSPVAXA,USB3,0,51.0,FINESTEERING,2107,283865.400,02000000,471d,15824;INS_ALIGNMENT_COMPLETE,INS_RTKFIXED,37.37071856255,126.72139199889,8.7824,22.3000,-0.5108,-0.3655,0.0313,-0.933274123,1.127883317,213.366579134,0.4336,0.3023,0.5928,0.1148,0.0954,0.0839,0.0963,0.1002,5.1456,0f000001,0*e5b04468\n\t", "INSPVAXA,USB3,0,51.0,FINESTEERING,2107,283865.900,02000000,471d,15824;INS_ALIGNMENT_COMPLETE,INS_RTKFIXED,37.37071661051,126.72139019548,8.7866,22.3000,-0.2777,-0.2015,0.0278,-1.149054728,0.648107164,213.765006412,0.4336,0.3023,0.5928,0.1148,0.0954,0.0839,0.0963,0.1002,5.1456,0f000001,0*0fe651af\n\t", "INSPVAXA,USB3,0,51.0,FINESTEERING,2107,283866.400,02000000,471d,15824;INS_ALIGNMENT_COMPLETE,INS_RTKFIXED,37.37071495847,126.72138864071,8.7911,22.3000,-0.4383,-0.3177,0.0305,-1.188306881,0.667471315,213.730398031,0.4343,0.3039,0.5934,0.1144,0.0951,0.0843,0.0964,0.1003,5.1466,0f000001,0*5b447a13\n\t", "INSPVAXA,USB3,0,51.0,FINESTEERING,2107,283866.900,02000000,471d,15824;INS_ALIGNMENT_COMPLETE,INS_RTKFIXED,37.37071327557,126.72138707282,8.7965,22.3000,-0.3634,-0.2672,0.0089,-1.371908474,0.653216644,213.825388529,0.4343,0.3039,0.5934,0.1144,0.0951,0.0843,0.0964,0.1003,5.1466,0f000001,0*b2617258\n\t", "INSPVAXA,USB3,0,52.0,FINESTEERING,2107,283867.400,02000000,471d,15824;INS_ALIGNMENT_COMPLETE,INS_RTKFIXED,37.37071150650,126.72138537987,8.7986,22.3000,-0.3586,-0.2741,0.0372,-1.171252823,0.553114037,213.926060837,0.4346,0.3035,0.5942,0.1136,0.0954,0.0837,0.0964,0.1003,5.1472,0f000001,0*449ce9b9\n\t", "INSPVAXA,USB3,0,52.0,FINESTEERING,2107,283867.900,02000000,471d,15824;INS_ALIGNMENT_COMPLETE,INS_RTKFIXED,37.37070986171,126.72138379312,8.8042,22.3000,-0.3895,-0.2987,0.0305,-0.968121893,0.950264581,213.826020130,0.4346,0.3035,0.5942,0.1136,0.0954,0.0837,0.0964,0.1003,5.1472,0f000001,0*7d4cf138\n\t", "INSPVAXA,USB3,0,53.5,FINESTEERING,2107,283868.400,02000000,471d,15824;INS_ALIGNMENT_COMPLETE,INS_RTKFIXED,37.37070816169,126.72138212704,8.8085,22.3000,-0.3715,-0.2818,0.0239,-0.767361494,1.034807260,213.960421110,0.4345,0.3021,0.5949,0.1138,0.0953,0.0840,0.0965,0.1004,5.1465,0f000001,
